vi "Initialize Attributes.vi"(8 "error in (no error)":errorcluster, 10 "Attribute Data":variant, 11 "CS++DeviceActor in":refnum<class "CS++DeviceActor.lvclass">) -> (0 "error out":errorcluster, 2 "Found?":bool, 3 "CS++DeviceActor out":refnum<class "CS++DeviceActor.lvclass">)   [LabVIEW 2013, in "CS++DeviceActor.lvlib" / "CS++DeviceActor.lvclass"]
doc: "Initialize object attribute.\n\nUnique resources should be allocated elsewhere!"
uses:
  CS++DeviceActor.lvclass
  CS++BaseActor/CS++BaseActor.lvclass
  CS++BaseActor/CS++BaseActor.lvclass/CS++BaseActor.ctl
  Classes/CS++BaseClasses/Factory/CS++Factory.lvclass
  CS++DeviceActor.lvclass/CS++DeviceActor.ctl
  Libraries/Base/CS++Base.lvlib
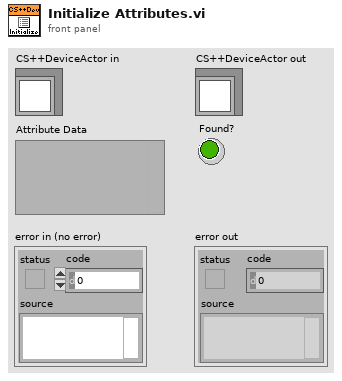
[diagram p1: front panel]
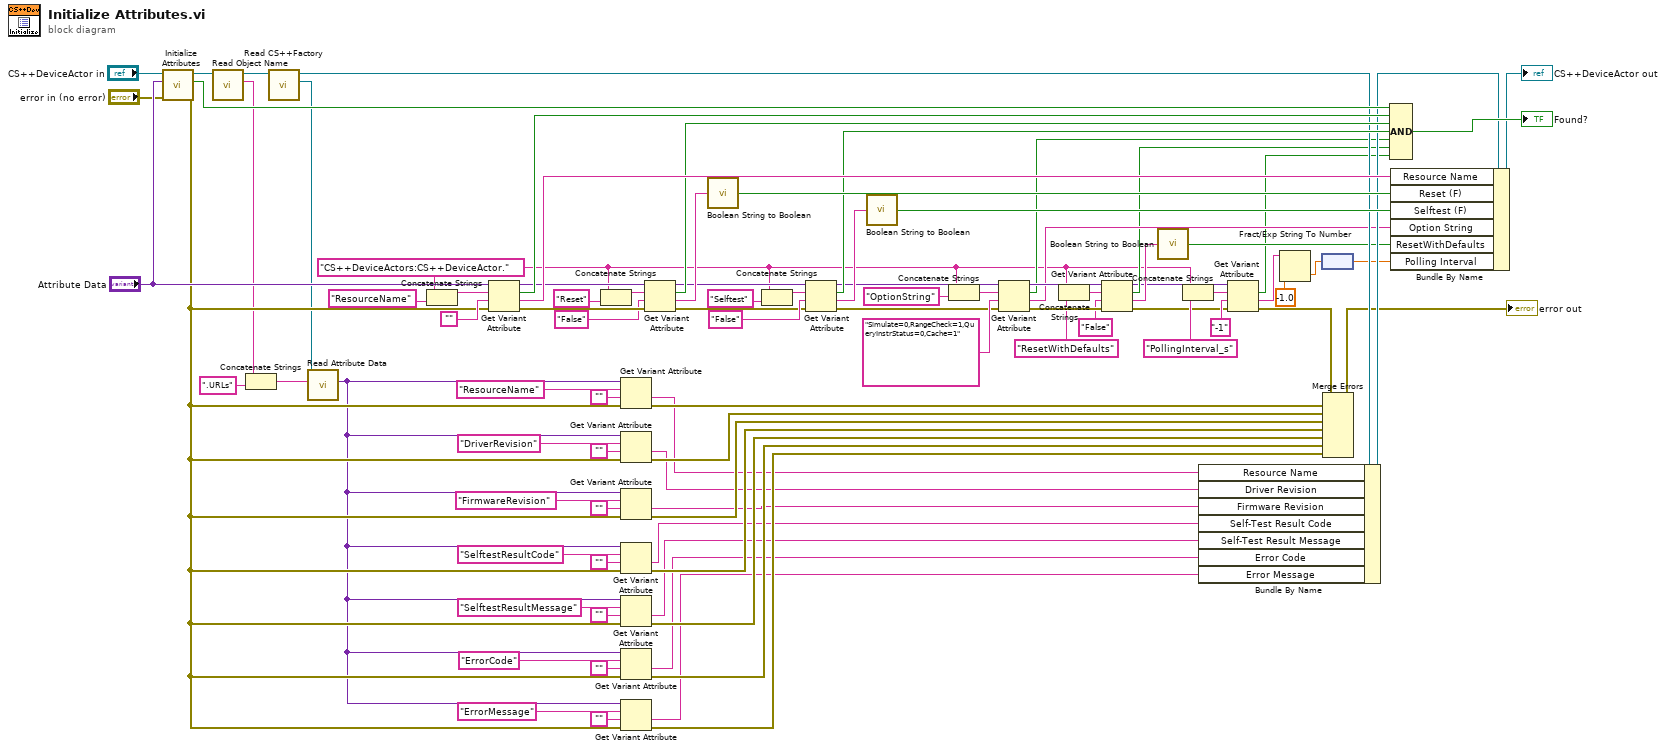
[diagram p0: block diagram]
diagram:
  w6 = "CS++DeviceActors:CS++DeviceActor."
  n1 = call-parent "Initialize Attributes.vi"("error in (no error)"="error in (no error)", "Attribute Data"="Attribute Data", "CS++BaseActor in"="CS++DeviceActor in") -> ("error out"=w70:errorcluster, "Found?"=w93:bool, "CS++BaseActor out"=w30:refnum<class "CS++DeviceActor.lvclass">)  [unwired: 6 in]
  n2 = call "Read Object Name.vi"("CS++BaseActor in"=w30) -> ("Object Name"=w43:string, "CS++BaseActor out"=w44:refnum<class "CS++DeviceActor.lvclass">)  [unwired: 8 in, 1 out]
  n3 = Concatenate Strings(w43, ".URLs" ("string")) -> (w41:string)
  n4 = call "Read CS++Factory.vi"("CS++BaseActor in"=w44) -> ("CS++Factory"=w45:refnum<class "CS++Factory.lvclass">, "CS++BaseActor out"=w32:refnum<class "CS++DeviceActor.lvclass">)  [unwired: 8 in, 1 out]
  n5 = call-dynamic "Read Attribute Data.vi"("Object Name"=w41, "CS++Factory in"=w45) -> ("Attribute Data"=w40:variant)  [unwired: 7 in, 2 out]
  n6 = Concatenate Strings(w6, "ResourceName") -> (w92:string)
  n7 = Get Variant Attribute(Variant="Attribute Data", name=w92, default value (empty Variant)="", error in=w70) -> (duplicate Variant=w84:variant, found=w87:bool, value=w89:string, error out=w83:errorcluster)
  n8 = Concatenate Strings(w6, "Reset") -> (w85:string)
  n9 = Get Variant Attribute(Variant=w40, name="ResourceName", default value (empty Variant)="", error in=w70) -> (value=w62:string, error out=w69:errorcluster)  [unwired: 2 out]
  n10 = Get Variant Attribute(Variant=w40, name="DriverRevision", default value (empty Variant)="", error in=w70) -> (value=w61:string, error out=w68:errorcluster)  [unwired: 2 out]
  n11 = Get Variant Attribute(Variant=w40, name="FirmwareRevision", default value (empty Variant)="", error in=w70) -> (value=w60:string, error out=w67:errorcluster)  [unwired: 2 out]
  n12 = Get Variant Attribute(Variant=w40, name="SelftestResultCode", default value (empty Variant)="", error in=w70) -> (value=w59:string, error out=w66:errorcluster)  [unwired: 2 out]
  n13 = Get Variant Attribute(Variant=w40, name="SelftestResultMessage", default value (empty Variant)="", error in=w70) -> (value=w58:string, error out=w65:errorcluster)  [unwired: 2 out]
  n14 = Get Variant Attribute(Variant=w40, name="ErrorCode", default value (empty Variant)="", error in=w70) -> (value=w57:string, error out=w64:errorcluster)  [unwired: 2 out]
  n15 = Get Variant Attribute(Variant=w40, name="ErrorMessage", default value (empty Variant)="", error in=w70) -> (value=w56:string, error out=w63:errorcluster)  [unwired: 2 out]
  n16 = Get Variant Attribute(Variant=w84, name=w85, default value (empty Variant)="False", error in=w83) -> (duplicate Variant=w53:variant, found=w79:bool, value=w81:string, error out=w47:errorcluster)
  n17 = call "Boolean String to Boolean.vi"("T/F String"=w81) -> ("Value"=w80:bool)
  n18 = Concatenate Strings(w6, "Selftest") -> (w55:string)
  n19 = Get Variant Attribute(Variant=w53, name=w55, default value (empty Variant)="False", error in=w47) -> (duplicate Variant=w18:variant, found=w49:bool, value=w52:string, error out=w13:errorcluster)
  n20 = call "Boolean String to Boolean.vi"("T/F String"=w52) -> ("Value"=w51:bool)
  n21 = Concatenate Strings(w6, "OptionString" ("string")) -> (w27:string)
  n22 = Get Variant Attribute(Variant=w18, name=w27, default value (empty Variant)="Simulate=0,RangeCheck=1,QueryInstrStatus=0,Cache=1" ("string"), error in=w13) -> (duplicate Variant=w23:variant, found=w15:bool, value=w16:string, error out=w24:errorcluster)
  n23 = Concatenate Strings(w6, "ResetWithDefaults" ("string")) -> (w22:string)
  n24 = Get Variant Attribute(Variant=w23, name=w22, default value (empty Variant)="False" ("string"), error in=w24) -> (duplicate Variant=w7:variant, found=w14:bool, value=w20:string, error out=w8:errorcluster)
  n25 = call "Boolean String to Boolean.vi"("T/F String"=w20) -> ("Value"=w17:bool)
  n26 = Concatenate Strings(w6, "PollingInterval_s" ("string")) -> (w10:string)
  n27 = Bundle By Name(cluster=w32, "Resource Name"=w62, "Driver Revision"=w61, "Firmware Revision"=w60, "Self-Test Result Code"=w59, "Self-Test Result Message"=w58, "Error Code"=w57, "Error Message"=w56) -> (w46:refnum<class "CS++DeviceActor.lvclass">)
  n28 = Get Variant Attribute(Variant=w7, name=w10, default value (empty Variant)="-1" ("string"), error in=w8) -> (found=w4:bool, value=w5:string, error out=w9:errorcluster)  [unwired: 1 out]
  n29 = Fract/Exp String To Number(string=w5, default (0 dbl)=-1.0 ("default (0 DBL)")) -> (number=w2:dbl)  [unwired: 2 in, 1 out]
  n30 = node(w2) -> (w1:dbl[unit])
  n31 = Merge Errors(w9, w69, w68, w67, w66, w65, w64, w63) -> (→"error out":errorcluster)
  n32 = Compound Arithmetic op=AND(w93, w87, w79, w49, w15, w14, w4) -> (→"Found?":bool)
  n33 = Bundle By Name(cluster=w46, "Resource Name"=w89, "Reset (F)"=w80, "Selftest (F)"=w51, "Option String"=w16, "ResetWithDefaults"=w17, "Polling Interval"=w1) -> (→"CS++DeviceActor out":refnum<class "CS++DeviceActor.lvclass">)
